vi "Timmer.vi"(5 "Seg RST 2":u16, 6 "Time has elapsed?":bool, 7 "Set stepps":u16) -> (2 "ok":bool, 3 "Seg RST":u16)   [LabVIEW 2021]
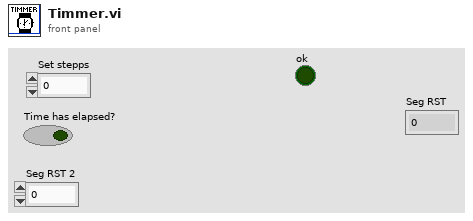
[diagram p1: front panel]
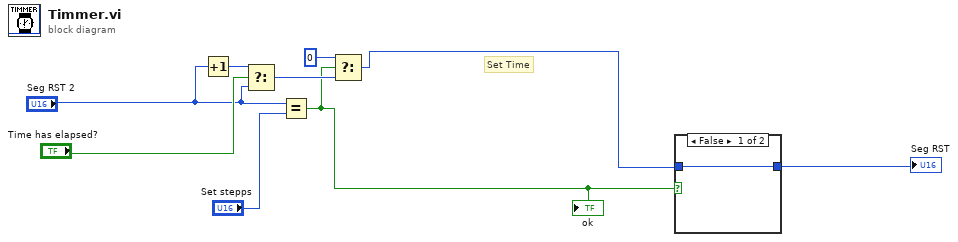
[diagram p0: block diagram]
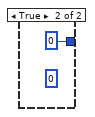
[diagram p2: hidden frame]
diagram:
  # "Set Time"
  n1 = Increment(x="Seg RST 2") -> (x+1=w9:u16)
  n2 = Select(t=w9, s="Time has elapsed?", f="Seg RST 2") -> (s? t:f=w7:u16)
  n3 = Equal?(x="Seg RST 2", y="Set stepps") -> (x = y?=w3:bool)
  "ok" <- w3
  n4 = Select(t=u16 0, s=w3, f=w7) -> (s? t:f=w4:u16)
  n5 = case shown="False" w3 {
    tunnel: w4 -> [w10 _]
    tunnel: [w10 u16 0 ("Min")] -> w6
    frame False {
    }
    frame True {
      (unwired) u16 0 ("S")
    }
  }
  "Seg RST" <- w6
